vi "Generate Simulated Data.vi"(8 "error in (no error)":cluster{"状态":bool, "代码":i32, "源":string} caption="错误输入（无错误）", 11 "信号类型":T1) -> (0 "error out":cluster{"状态":bool, "代码":i32, "源":string} caption="错误输出", 2 "图形数据":waveform(dbl)[](array[waveform]))   [LabVIEW 2018, in "Acquisition.lvlib"]
doc: "按硬件配置输入中的信号类型，生成采样波形。"
uses:
  Acquisition.lvlib
  Signal Type.ctl
  <vilib>/measure/NI_MABase.lvlib
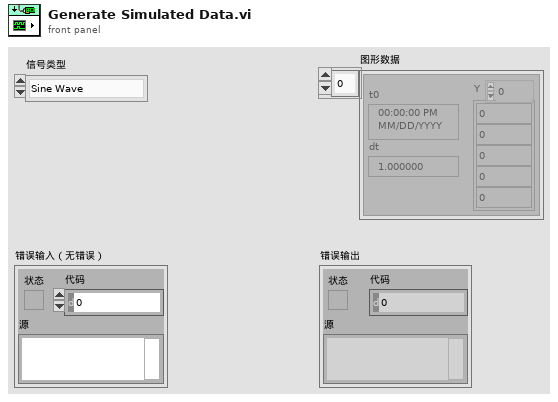
[diagram p1: front panel]
types:
  T1 = typedef "Acquisition.lvlib/Signal Type.ctl" = enum16{"Sine Wave", "Square with Noise"}
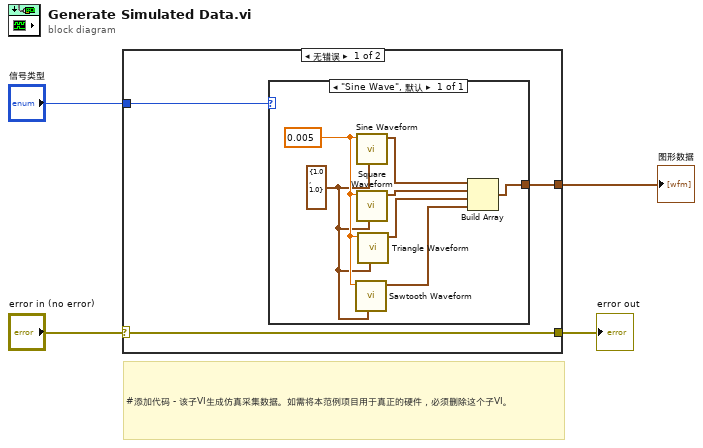
[diagram p0: block diagram]
diagram:
  # "#添加代码 - 该子VI生成仿真采集数据。如需将本范例项目用于真正的硬件，必须删除这个子VI。"
  n1 = case shown="无错误" "error in (no error)" {
    selector: "error in (no error)" -> [w7 w15]
    tunnel: [w7 w15] -> w3
    tunnel: "信号类型" -> [w6 _]
    tunnel: [w5 _] -> w1
    frame No Error {
      n2 = case shown="\"Sine Wave\", 默认" w6 {
        tunnel: [w14] -> w5
        frame "Sine Wave", Default {
          w8 = cluster{"Fs":dbl, "#s":dbl} {"Fs"=1.0, "#s"=1.0} ("sampling info")
          w13 = 0.005 ("frequency")
          n3 = call <vilib>:"Sawtooth Waveform.vi"("sampling info"=w8, "frequency"=w13) -> ("signal out"=w12:waveform(dbl))  [unwired: 8 in, 1 out]
          n4 = call <vilib>:"Sine Waveform.vi"("sampling info"=w8, "frequency"=w13) -> ("signal out"=w9:waveform(dbl))  [unwired: 8 in, 1 out]
          n5 = call <vilib>:"Square Waveform.vi"("sampling info"=w8, "frequency"=w13) -> ("signal out"=w10:waveform(dbl))  [unwired: 8 in, 1 out]
          n6 = call <vilib>:"Triangle Waveform.vi"("sampling info"=w8, "frequency"=w13) -> ("signal out"=w11:waveform(dbl))  [unwired: 8 in, 1 out]
          n7 = Build Array(w9, w10, w11, w12) -> (w14:waveform(dbl)[])
        }
      }
    }
    frame Error {
    }
  }
  "error out" <- w3
  "图形数据" <- w1
